vi "Read Device.vi"(8 "error in (no error)":errorcluster, 11 "Launch Hardware Settings Msg in":refnum<class "Launch Hardware Settings Msg.lvclass">) -> (0 "error out":errorcluster, 2 "Device":i32, 3 "Launch Hardware Settings Msg out":refnum<class "Launch Hardware Settings Msg.lvclass">)   [LabVIEW 2017, in "Measurement UI.lvlib" / "Launch Hardware Settings Msg.lvclass"]
uses:
  Launch Hardware Settings Msg.lvclass
  Launch Hardware Settings Msg.lvclass/Launch Hardware Settings Msg.ctl
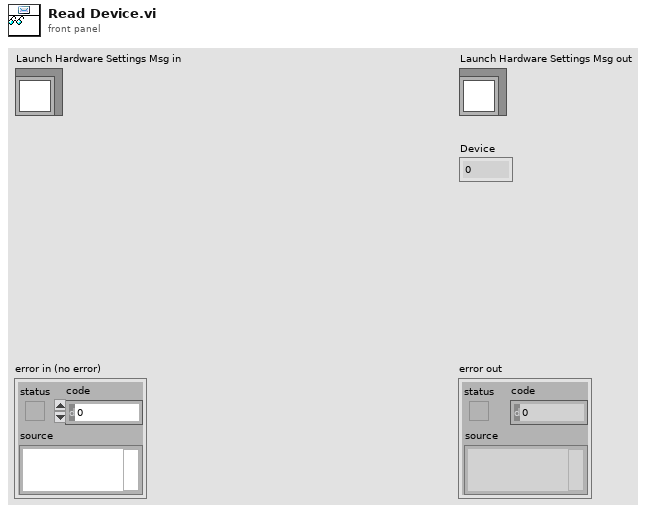
[diagram p1: front panel]
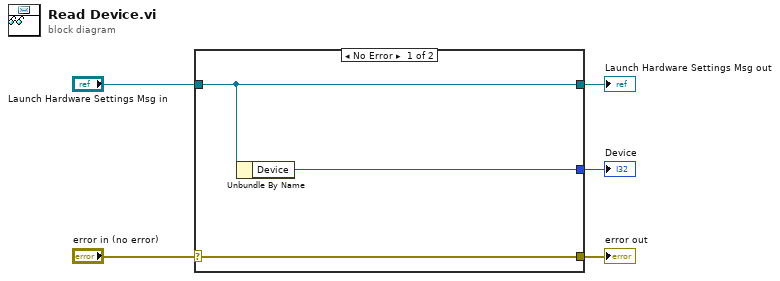
[diagram p0: block diagram]
diagram:
  n1 = case shown="No Error" "error in (no error)" {
    selector: "error in (no error)" -> [w8 w9]
    tunnel: [w8 w9] -> w4
    tunnel: [w7 w10] -> w2
    tunnel: "Launch Hardware Settings Msg in" -> [w7 w10]
    tunnel: [w6 _] -> w1
    frame No Error {
      n2 = Unbundle By Name(w7) -> ("Device"=w6:i32)
    }
    frame Error {
    }
  }
  "error out" <- w4
  "Launch Hardware Settings Msg out" <- w2
  "Device" <- w1
